vi "Seq-Globals.vi"() -> ()   [LabVIEW 2020]
panel:
  in  "Allow advanced":bool
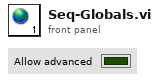
[diagram p1: front panel]
diagram:
